vi "NO-1_10Hz_RW.vi"(8 "Timeout (ms)":u32=50, 9 "TimeoutW (ms)":i32=1, 10 "TimeoutR (ms)":i32=10, 11 "Byte Array":u8[](array[numeric])=[65, 48, 48, 48, 48, 48, 13]) -> (0 "Fault":bool, 3 "MFC out":u8[](array[numeric]))   [LabVIEW 2014]
uses:
  <vilib>/rvi/Emulation/niFpgaGetClockAttributes.vi
  <vilib>/rvi/Emulation/niFpgaSctlEmulationGetInTimedLoop.vi
  <vilib>/rvi/Emulation/niFpgaEmulationReportErrorSimple.vi
  <vilib>/rvi/eio/common/nirviEmuTemplateMethod_errors.vi
  <vilib>/rvi/Emulation/niFpgaCriticalErrorInLSC.vi
  <vilib>/eio/EIOMethodNode/EIOMethodNode.xnode
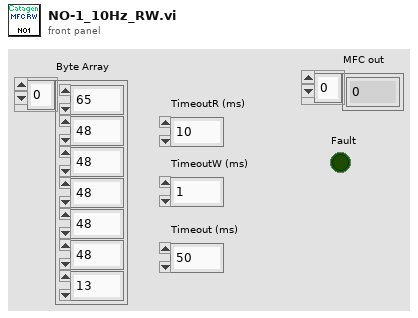
[diagram p1: front panel]
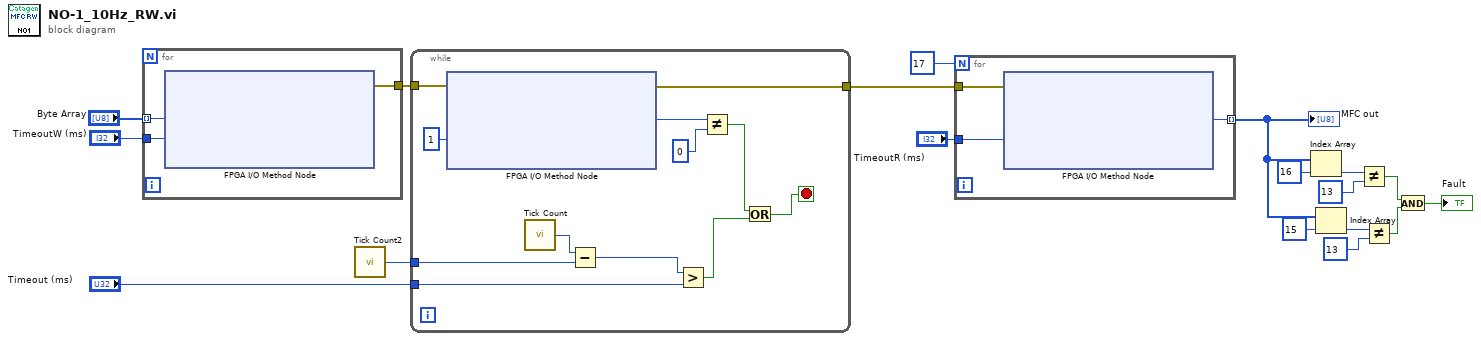
[diagram p0: block diagram]
diagram:
  n1 = for {
    tunnel: "Byte Array" -> [w21] mode=indexing
    tunnel: [w20] -> w16
    tunnel: "TimeoutW (ms)" -> [w19]
    n2 = xnode "FPGA I/O Method Node"("Data"=w21, "Timeout (ms)"=w19) -> ("error out"=w20:errorcluster)  [unwired: 2 in, 2 out]
  }
  n3 = call "Tick Count2"() -> ("Tick Count(mSec)"=w8:u32)
  n4 = while {
    tunnel: w16 -> [w33]
    tunnel: [w29] -> w13
    tunnel: "Timeout (ms)" -> [w23]
    tunnel: w8 -> [w22]
    stop <- w24 stop-if-true
    n5 = xnode "FPGA I/O Method Node"("error in"=w33, "Timeout (ms)"=1) -> ("error out"=w29:errorcluster, "Data"=w31:u8)  [unwired: 1 in, 2 out]
    n6 = call "Tick Count"() -> ("Tick Count(mSec)"=w26:u32)
    n7 = Subtract(x=w26, y=w22) -> (x-y=w27:u32)
    n8 = Greater?(x=w27, y=w23) -> (0:w28:bool)
    n9 = Not Equal?(x=w31, y=u8 0) -> (x != y?=w25:bool)
    n10 = Or(x=w25, y=w28) -> (x .or. y?=w24:bool)
  }
  n11 = for {
    N: 17 -> [_]
    tunnel: w13 -> [w36]
    tunnel: [w35] -> w4 mode=indexing
    tunnel: "TimeoutR (ms)" -> [w34]
    n12 = xnode "FPGA I/O Method Node"("error in"=w36, "Timeout (ms)"=w34) -> ("Data"=w35:u8)  [unwired: 1 in, 3 out]
  }
  "MFC out" <- w4
  n13 = Index Array(array=w4, index=16) -> (element=w11:u8)
  n14 = Index Array(array=w4, index=15) -> (element=w6:u8)
  n15 = Not Equal?(x=w11, y=u8 13) -> (x != y?=w2:bool)
  n16 = Not Equal?(x=w6, y=u8 13) -> (x != y?=w1:bool)
  n17 = And(x=w2, y=w1) -> (x .and. y?=→"Fault":bool)
